vi "Actor Core.vi"(8 "error in":errorcluster, 11 "GRAFICAR_SEÑAL_ACTUALIZABLE in":refnum<class "GRAFICAR_SEÑAL_ACTUALIZABLE.lvclass">) -> (0 "error out":errorcluster, 3 "Actor out":refnum<class "Actor.lvclass">)   [LabVIEW 2019, in "GRAFICAR_SEÑAL_ACTUALIZABLE.lvlib" / "GRAFICAR_SEÑAL_ACTUALIZABLE.lvclass"]
doc: "(<B>Filename</B>: Actor Framework.lvlib:Actor.lvclass:Actor Core.vi)\n\nReceives messages to the actor, reacts to them, and initiates any error handling that may shut the actor down.\n\nDescendant classes may override this VI to append parallel tasks for the actor to complete while it handles messages. Overrides use the Call Parent Method node."
uses:
  C:/Program Files (x86)/National Instruments/LabVIEW 2019/vi.lib/ActorFramework/Actor/Actor.lvclass
  <vilib>/ActorFramework/Actor/Actor.lvclass
  <vilib>/ActorFramework/Actor/Actor.lvclass/Actor.ctl
  <vilib>/ActorFramework/Message Enqueuer/Message Enqueuer.lvclass/Message Enqueuer.ctl
  <vilib>/ActorFramework/Message Enqueuer/Enqueue.vi
  C:/Program Files (x86)/National Instruments/LabVIEW 2019/vi.lib/ActorFramework/Message/Message.lvclass
  <vilib>/ActorFramework/Message Priority Queue/Priority Enqueue.vi
  <vilib>/measure/NI_MABase.lvlib
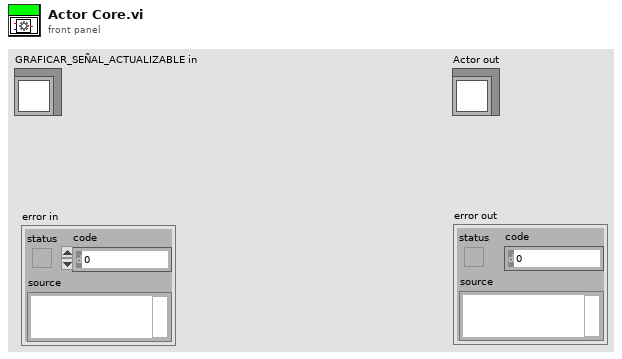
[diagram p1: front panel]
types:
  T1 = cluster{"signal type":enum16{"Sine Wave", "Triangle Wave", "Square Wave", "Sawtooth Wave"}, "amplitude":dbl, "frequency":dbl}
  T2 = cluster{"START/STOP HL":refnum<user-event>, "EXIT":refnum<user-event>, "PARÁMETROS":refnum<user-event>}
  T3 = enum16{"Sine Wave", "Triangle Wave", "Square Wave", "Sawtooth Wave"}
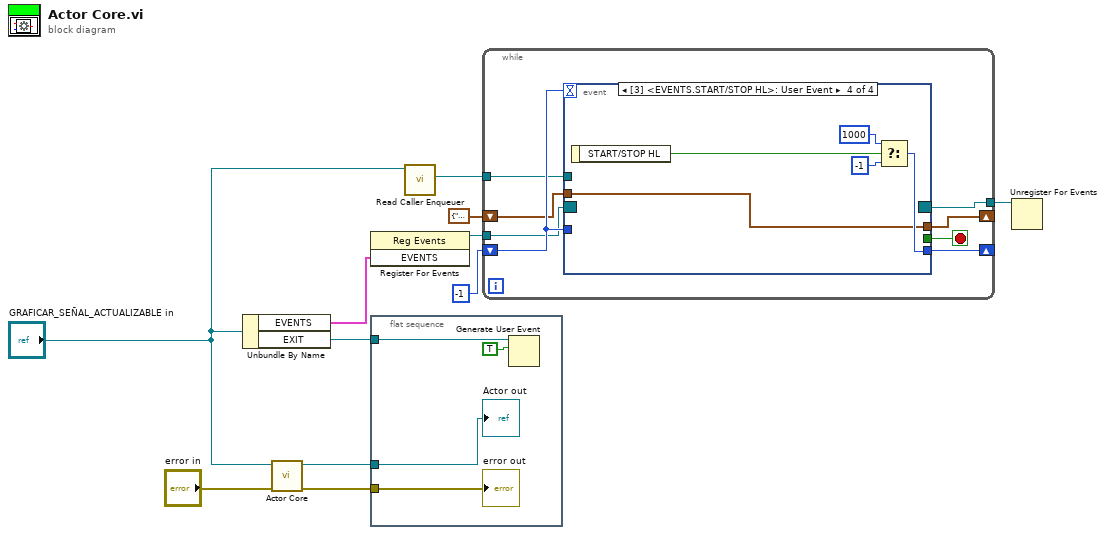
[diagram p0: block diagram]
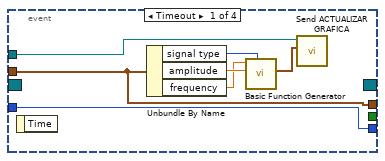
[diagram p2: hidden frame]
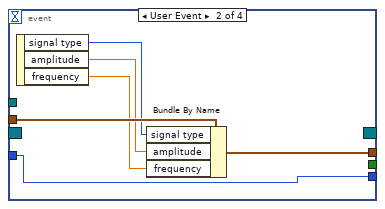
[diagram p3: hidden frame]
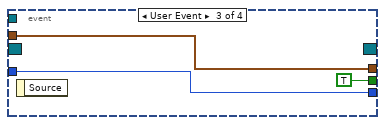
[diagram p4: hidden frame]
diagram:
  n1 = Unbundle By Name("GRAFICAR_SEÑAL_ACTUALIZABLE in") -> ("EVENTS"=w7:T2, "EXIT"=w4:refnum<user-event>)
  n2 = call-parent "Actor Core.vi"("error in"="error in", "Actor in"="GRAFICAR_SEÑAL_ACTUALIZABLE in") -> ("error out"=w11:errorcluster, "Actor out"=w10:refnum<class "Actor.lvclass">)  [unwired: 8 in]
  n3 = register-events(w7) -> (reference out=w6:refnum<event-registration>)  [unwired: 2 in, 1 out]
  n4 = flat-sequence {
    tunnel: w11 -> [w15]
    tunnel: w10 -> [w14]
    tunnel: w4 -> [w13]
    frame #0 {
      n5 = Generate User Event(user event=w13, event data cluster=TRUE ("event data")) -> ()  [unwired: 2 in, 2 out]
      "error out" <- w15
      "Actor out" <- w14
    }
  }
  n6 = call <vilib>:"Read Caller Enqueuer.vi"("Actor"="GRAFICAR_SEÑAL_ACTUALIZABLE in") -> ("Caller Enqueuer"=w1:refnum<class "Message Enqueuer.lvclass">)  [unwired: 10 in]
  n7 = while {
    shift-right: [w22] -> _
    shift-left: -1 -> [w23]
    tunnel: w6 -> [w21]
    tunnel: [w20] -> w5
    shift-right: [w17] -> _
    shift-left: T1 {"signal type"=enum."Sine Wave", "amplitude"=0.0, "frequency"=0.0} -> [w18]
    tunnel: w1 -> [w16]
    stop <- w19 stop-if-true
    n8 = event shown="[3] <EVENTS.START/STOP HL>: User Event" {
      selector: w21 -> [_ _ _ _]
      dyn-events: [_ _ _ _] -> w20
      timeout: w23 -> [_ _ _ _]
      tunnel: w23 -> [w30 w31 w37 _]
      tunnel: [w30 w31 w37 w41] -> w22
      tunnel: [_ _ TRUE _] -> w19
      tunnel: w18 -> [w24 w36 w38 w40]
      tunnel: [w24 w32 w38 w40] -> w17
      tunnel: w16 -> [w25 _ _ _]
      event Timeout {
        n9 = event-data() -> ()  [unwired: 1 in, 1 out]
        n10 = Unbundle By Name(w24) -> ("signal type"=w29:T3, "amplitude"=w28:dbl, "frequency"=w27:dbl)
        n11 = call <vilib>:"Basic Function Generator.vi"("signal type"=w29, "amplitude"=w28, "frequency"=w27) -> ("signal out"=w26:waveform(dbl))  [unwired: 6 in, 2 out]
        n12 = call "Send ACTUALIZAR GRAFICA.vi"("event data"=w26, "Message Enqueuer"=w25) -> ()  [unwired: 8 in, 2 out]
      }
      event User Event {
        n13 = event-data() -> ("signal type"=w35:T3, "amplitude"=w34:dbl, "frequency"=w33:dbl)  [unwired: 1 in]
        n14 = Bundle By Name(cluster=w36, "signal type"=w35, "amplitude"=w34, "frequency"=w33) -> (w32:T1)
      }
      event User Event {
        n15 = event-data() -> ()  [unwired: 1 in, 1 out]
      }
      event User Event {
        n16 = event-data() -> ("START/STOP HL"=w44:bool)  [unwired: 1 in]
        n17 = Select(t=1000, s=w44, f=-1) -> (s? t:f=w41:i32)
      }
    }
  }
  n18 = Unregister For Events(event registration refnum=w5) -> ()  [unwired: 1 in, 1 out]
